vi "TCP Test.vi"() -> ()   [LabVIEW 2017]
panel:
  in  "Start / Abort Button":bool
  in  "stop":bool
  out "data out":string
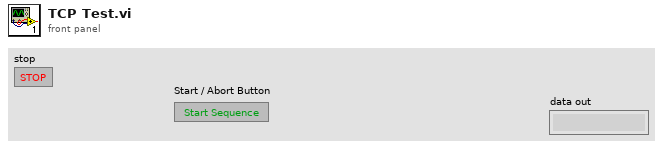
[diagram p1: front panel]
types:
  T1 = enum16{"Standard", "Buffered", "CRLF", "Immediate"}
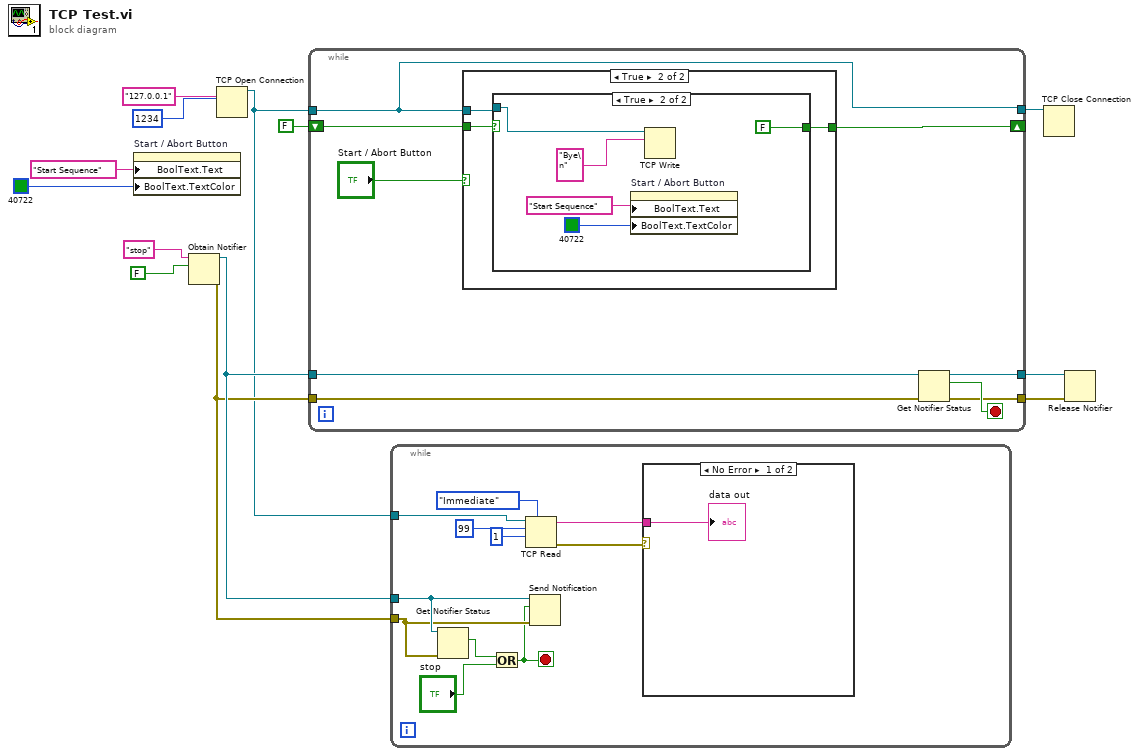
[diagram p0: block diagram]
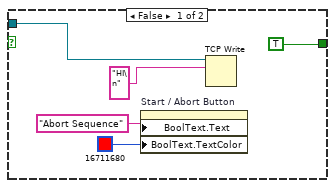
[diagram p3: hidden frame]
diagram:
  n1 = property on="Start / Abort Button" class="Bool"("BoolText.Text"="Start Sequence" ("Boolean Text.Text"), "BoolText.TextColor"=u32 40722) -> ()  [unwired: 2 in, 2 out]
  n2 = Obtain Notifier(name (unnamed)="stop", notification data type=FALSE) -> (notifier out=w9:refnum<notifier>, error out=w8:errorcluster)  [unwired: 2 in, 1 out]
  n3 = TCP Open Connection(address="127.0.0.1", remote port or service name=u16 1234) -> (connection ID=w5:refnum<k5>)  [unwired: 3 in, 1 out]
  n4 = while {
    tunnel: w9 -> [w22]
    tunnel: w8 -> [w21]
    tunnel: [w19] -> w7
    tunnel: [w18] -> w6
    tunnel: w5 -> [w17]
    tunnel: [w17] -> w4
    shift-right: [w16] -> _
    shift-left: FALSE -> [w15]
    stop <- w20 stop-if-true
    n5 = case shown="True" "Start / Abort Button" {
      tunnel: w17 -> [_ w26]
      tunnel: [w23 w25] -> w16
      tunnel: w15 -> [w23 w24]
      frame False {
      }
      frame True {
        n6 = case shown="True" w24 {
          tunnel: w26 -> [w29 w35]
          tunnel: [TRUE FALSE] -> w25
          frame False {
            n7 = property on="Start / Abort Button" class="Bool"("BoolText.Text"="Abort Sequence" ("Boolean Text.Text"), "BoolText.TextColor"=u32 16711680) -> ()  [unwired: 2 in, 2 out]
            n8 = TCP Write(connection ID=w29, data in="HI\n") -> ()  [unwired: 2 in, 3 out]
          }
          frame True {
            n9 = property on="Start / Abort Button" class="Bool"("BoolText.Text"="Start Sequence" ("Boolean Text.Text"), "BoolText.TextColor"=u32 40722) -> ()  [unwired: 2 in, 2 out]
            n10 = TCP Write(connection ID=w35, data in="Bye\n") -> ()  [unwired: 2 in, 3 out]
          }
        }
      }
    }
    n11 = Get Notifier Status(notifier=w22, error in (no error)=w21) -> (notifier out=w19:refnum<notifier>, current notification=w20:bool, error out=w18:errorcluster)  [unwired: 2 out]
  }
  n12 = while {
    tunnel: w5 -> [w42]
    tunnel: w9 -> [w41]
    tunnel: w8 -> [w40]
    stop <- w37 stop-if-true
    n13 = Get Notifier Status(notifier=w41, error in (no error)=w40) -> (current notification=w39:bool)  [unwired: 4 out]
    n14 = Or(x=w39, y="stop") -> (x .or. y?=w37:bool)
    n15 = TCP Read(connection ID=w42, bytes to read=99, 7:T1."Immediate" ("mode (standard)"), 9:1 ("timeout ms (25000)")) -> (data out=w47:string, error out=w46:errorcluster)  [unwired: 1 in, 1 out]
    n16 = Send Notification(notification=w37, notifier=w41, error in (no error)=w40) -> ()  [unwired: 2 out]
    n17 = case shown="No Error" w46 {
      tunnel: w47 -> [w48 _]
      frame No Error {
        "data out" <- w48
      }
      frame Error {
      }
    }
  }
  n18 = TCP Close Connection(connection ID=w4) -> ()  [unwired: 2 in, 2 out]
  n19 = Release Notifier(notifier=w7, error in (no error)=w6) -> ()  [unwired: 1 in, 3 out]
